vi "Teleop.vi"(10 "Match Info":T2={"Autonomous Elapsed Seconds"=0.0, "TeleOp Elapsed Seconds"=0.0, "Disabled Elapsed Seconds"=0.0, "Visited Autonomous"=FALSE, "Visited TeleOp"=FALSE, "Visited Disabled"=FALSE, "Autonomous Settings"={"Autonomous Style"=enum."Independent", "VI Refnum"=refnum}}, 11 "Call Context":T3) -> ()   [LabVIEW 2013]
doc: "This VI is called for each TeleOp packet received from the DS where the robot is not disabled. It is often used to read from the joysticks and update I/O or to update setpoints for timed control loops. It should complete and return within 20 milliseconds or it may miss DS packets."
uses:
  <vilib>/Rock Robotics/WPI/DriverStation/WPI_DriverStationDerivedRobotMode.ctl
  <vilib>/Rock Robotics/WPI/DriverStation/WPI_DriverStationMatch Info.ctl
  <vilib>/Rock Robotics/WPI/Joystick/WPI_JoystickButtonState.ctl
  <vilib>/Rock Robotics/WPI/DriverStation/WPI_DriverStationRobotMode2.ctl
  Robot Global Data.vi
  <vilib>/Rock Robotics/WPI/Joystick/WPI_JoystickGetSetRefNum.vi
  <vilib>/Rock Robotics/WPI/RobotDrive/WPI_RobotDriveGetSetRefNum.vi
  <vilib>/addons/control/pid/pid.llb/PID Control Input Filter (DBL).vi
  <vilib>/addons/control/pid/NI_PID_pid.lvlib
panel:
  in  "Drive Controls":T1
  in  "Azimuth Enabled":bool
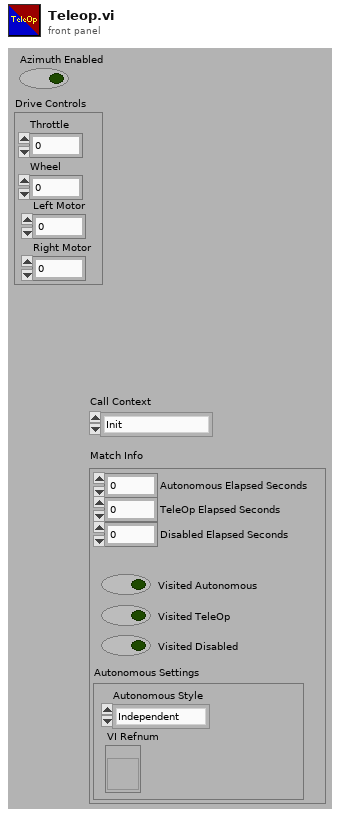
[diagram p1: front panel]
types:
  T1 = cluster{"Throttle":dbl, "Wheel":dbl, "Right Motor":dbl, "Left Motor":dbl}
  T2 = typedef "WPI_DriverStationMatch Info.ctl" = cluster{"Autonomous Elapsed Seconds":dbl, "TeleOp Elapsed Seconds":dbl, "Disabled Elapsed Seconds":dbl, "Visited Autonomous":bool, "Visited TeleOp":bool, "Visited Disabled":bool, "Autonomous Settings":cluster{"Autonomous Style":enum16{"Iterative", "Independent"}, "VI Refnum":refnum<vi>}}
  T3 = typedef "WPI_DriverStationDerivedRobotMode.ctl" = enum16{"Init", "Execute", "Stop"}
  T4 = typedef "WPI_JoystickButtonState.ctl" = cluster{"Button 1":bool, "Button 2":bool, "Button 3":bool, "Button 4":bool, "Button 5":bool, "Button 6":bool, "Button 7":bool, "Button 8":bool, "Button 9":bool, "Button 10":bool, "Button 11":bool, "Button 12":bool}
  T5 = cluster{"Driver Axes":cluster{"axis 1 (x)":dbl, "axis 2 (y)":dbl, "axis 3 (throttle)":dbl, "axis 4":dbl, "axis 5":dbl, "axis 6":dbl}, "Driver Buttons":T4, "Manipulator Axes":cluster{"axis 1 (x)":dbl, "axis 2 (y)":dbl, "axis 3 (throttle)":dbl, "axis 4":dbl, "axis 5":dbl, "axis 6":dbl}, "Manipulator Buttons":T4}
  T6 = typedef "WPI_JoystickDevRef.ctl" = cluster{"Device":T7}
  T7 = typedef "WPI_JoystickDeviceEnum.ctl" = enum16{"USB 1", "USB 2", "USB 3", "USB 4", "Kinect 1", "Kinect 2"}
  T8 = typedef "WPI_RobotDriveDevRef.ctl" = cluster{"DevStatus":errorcluster, "Motors[]":T9[], "Square Inputs":bool, "Max Output":dbl, "Isochronous":bool}
  T9 = typedef "WPI_MotorControlDeviceRef.ctl" = cluster{"DeviceStatus":errorcluster, "Type":enum16{"PWM", "CAN"}, "PWM":cluster{"Digital Module":T10, "PWM Channel":T11, "DeadBand":T12}, "CAN":cluster{"Device Number":u8, "Control Mode":T13, "Semaphore":T14, "Max Vout":dbl}, "Invert":bool, "TransformRef":T15, "InvTransformRef":T15}
  T10 = typedef "FPGA_TypedefDigitalModule.ctl" = enum16{"Digital Module 1", "Digital Module 2"}
  T11 = typedef "FPGA_DIOPWMChannel.ctl" = enum8{"PWM 1", "PWM 2", "PWM 3", "PWM 4", "PWM 5", "PWM 6", "PWM 7", "PWM 8", "PWM 9", "PWM 10", "Invalid"}
  T12 = typedef "WPI_PWMDeadband.ctl" = cluster{"Name":string, "maxPositivePwm":i32, "minPositivePwm":i32, "centerPwm":i32, "maxNegativePwm":i32, "minNegativePwm":i32, "angularRange":u16}
  T13 = typedef "WPI_CANJaguar_ControlMode.ctl" = enum8{"Percent VBus", "Current", "Speed", "Position", "Voltage"}
  T14 = typedef "Semaphore RefNum" = refnum<k1>
  T15 = typedef "WPI_PWMTransform_ConPane.ctl" = refnum<vi>
  T16 = cluster{"axis 1 (x)":dbl, "axis 2 (y)":dbl, "axis 3 (throttle)":dbl, "axis 4":dbl, "axis 5":dbl, "axis 6":dbl}
  T17 = enum16{"Wait", "Adjust Angle", "Warmup Shooter", "Fire", "Feeding", "Neutral Angle"}
  T18 = typedef "WPI_DriverStationRobotMode2.ctl" = enum16{"Autonomous Disabled", "Autonomous Enabled", "Teleop Disabled", "Teleop Enabled", "Timeout", "Finish", "Test Disabled", "Test Enabled"}
  T19 = cluster{"Quickturn_Sens_Low":dbl, "Quickturn_Sens_High":dbl, "Speedturn_Sens_Low":dbl, "Speedturn_Sens_High":dbl}
  T20 = cluster{"proportional gain (Kc)":dbl, "integral time (Ti, min)":dbl, "derivative time (Td, min)":dbl}
  T21 = typedef "Autonomous Commands.ctl" = cluster{"Load":bool, "Warmup":bool, "Low Gear":bool, "Shoot Angle":dbl, "Azimuth":bool, "Elevator":bool, "Neutral Angle":dbl, "Two Discs":bool, "Shoot":bool}
  T22 = typedef "UDP Dashboard Packet.ctl" = cluster{"Feed Angle":dbl, "Neutral Angle":dbl, "Autonomous Setpoints":T23, "Auto Shift":T24, "Elevator Angle Offset":dbl, "Potentiometer Angle":cluster{"Pot M":dbl, "Pot B":dbl}, "Shoot Setpoints":cluster{"Vision":T25, "Back Corner":T25, "Front":T25, "Front Corner":T25, "Half Court":T25, "Full Court":T25, "Pyramid":T25}, "Halo Drive":T26, "Auto Speed Constants":T27, "Shooting Delays":cluster{"Unjam On":dbl, "Unjam Off":dbl, "Flipper On":dbl, "Flipper Off":dbl, "Hopper Up":dbl}, "Left Roller Pwr":dbl, "Right Roller Pwr":dbl, "Elevator PID Gains":cluster{"proportional gain (Kc)":dbl, "integral time (Ti, min)":dbl, "derivative time (Td, min)":dbl}, "Elevator PID Output Range":cluster{"output high":dbl, "output low":dbl}, "Elevator Angle Tolerance":dbl, "Toggle Ears Delay":dbl, "Toggle Ears Distance":dbl, "Unjam Servo Angle":dbl, "Auton Steer PID gains":cluster{"proportional gain (Kc)":dbl, "integral time (Ti, min)":dbl, "derivative time (Td, min)":dbl}, "Auton Steer output range":cluster{"output high":dbl, "output low":dbl}, "Auto Reverse Speed":dbl, "Auto Stop Throttle":dbl, "Auto Stop Duration":dbl, "Spin output range":cluster{"output high":dbl, "output low":dbl}, "Spin PID gains":cluster{"proportional gain (Kc)":dbl, "integral time (Ti, min)":dbl, "derivative time (Td, min)":dbl}, "Auto-Center Line":T28, "Auton Distance PID gains Low Gear":cluster{"proportional gain (Kc)":dbl, "integral time (Ti, min)":dbl, "derivative time (Td, min)":dbl}, "Auton Distance output range":cluster{"output high":dbl, "output low":dbl}, "Auton Distance Threshold":dbl, "Auton Velocity Cutoff":dbl, "Auton Distance output range Center Line":cluster{"output high":dbl, "output low":dbl}, "Auton Distance PID gains High Gear":cluster{"proportional gain (Kc)":dbl, "integral time (Ti, min)":dbl, "derivative time (Td, min)":dbl}}
  T23 = typedef "Autonomous Setpoints.ctl" = cluster{"Shoot Angle 1":dbl, "Initial Delay":dbl, "Disc Count 1":dbl, "Shoot Time 1":dbl, "Distance 1":dbl, "Two Disc Distance 1":dbl, "Distance 2":dbl, "Two Disc Distance 2":dbl, "Distance 3":dbl, "Two Disc Distance 3":dbl, "Shoot Angle 3":dbl, "Disc Count 3":dbl, "Shoot Time 3":dbl, "Distance 4":dbl, "Two Disc Distance 4":dbl, "Low Gear":bool, "Shoot 1 Post Delay":dbl}
  T24 = typedef "Auto Shift Settings.ctl" = cluster{"Enabled":bool, "Upshift Speed":dbl, "Downshift Speed":dbl, "Upshift Throttle":dbl, "Turn Power Diff":dbl, "Motor Limit":dbl, "Encoder Limit":dbl}
  T25 = typedef "Shoot Profile.ctl" = cluster{"Pre RPM":dbl, "Main RPM":dbl, "Angle":dbl}
  T26 = typedef "Halo Drive.ctl" = cluster{"Gains":cluster{"Quickturn_Sens_Low":dbl, "Quickturn_Sens_High":dbl, "Speedturn_Sens_Low":dbl, "Speedturn_Sens_High":dbl}, "QuickTurn Const":dbl, "Loading Throttle Limit":dbl}
  T27 = typedef "Auto Speed Constants.ctl" = cluster{"Slowing Distance":dbl, "High Speed":dbl, "Rampup Time":dbl, "Low Speed":dbl, "High Speed (Reverse)":dbl}
  T28 = typedef "Autonomous Center Line Setpoints.ctl" = cluster{"Arc Turn x-axis":dbl, "Arc Turn y-axis":dbl, "Arc Turn Distance":dbl, "Distance 1":dbl, "Two Disc Distance 1":dbl, "Distance 2":dbl, "Two Disc Distance 2":dbl, "Spin Angle":dbl, "Spin Angle tolerance":dbl, "Spin y-axis":dbl, "Spin Distance":dbl, "Center Line Enabled":bool, "Distance 3":dbl, "Two Disc Distance 3":dbl, "Spin Angle 2":dbl, "Spin Angle tolerance 2":dbl, "Spin y-axis 2":dbl, "Spin Distance 2":dbl, "Shoot Angle 1":dbl, "Disc Count 1":dbl, "Shoot Time 1":dbl, "Shoot Angle 3":dbl, "Disc Count 3":dbl, "Shoot Time 3":dbl, "Low Gear":bool}
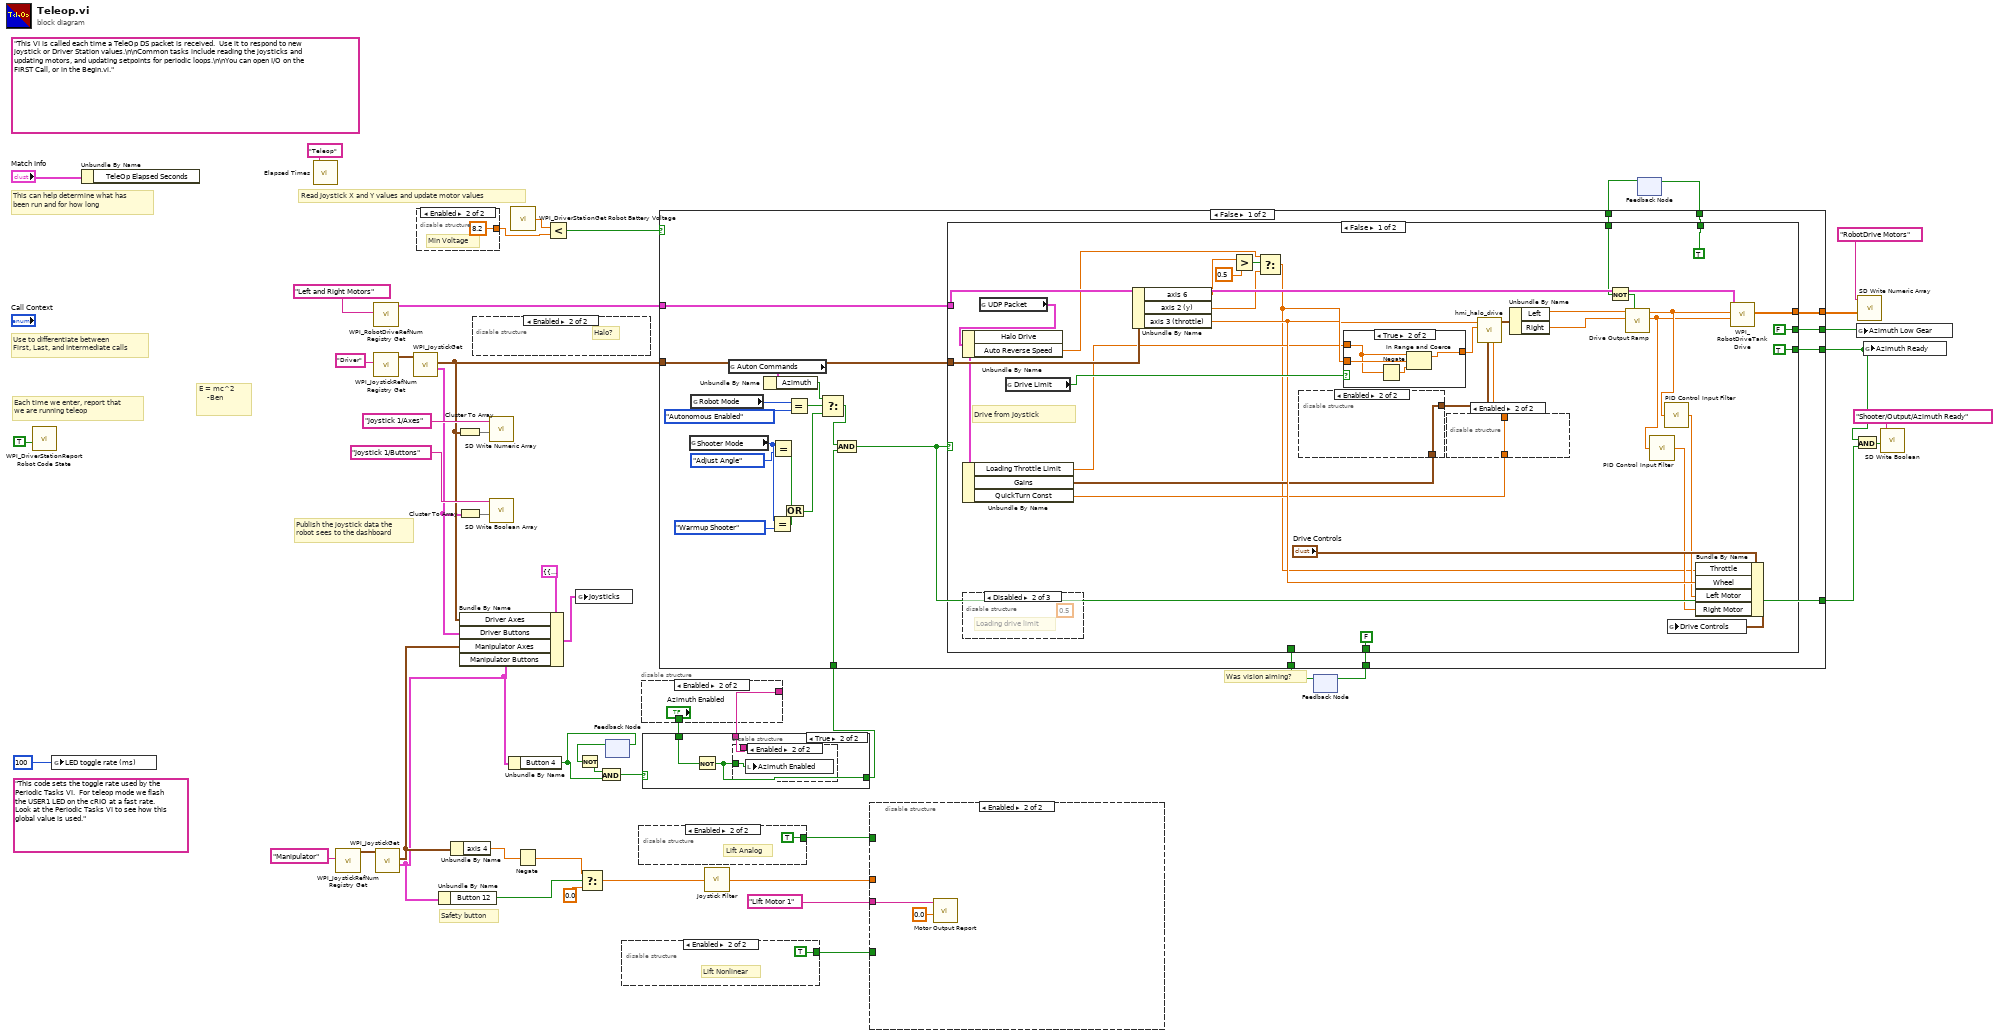
[diagram p0: block diagram]
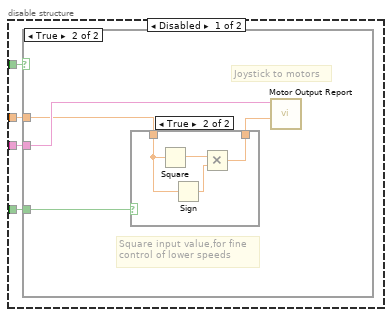
[diagram p2: hidden frame]
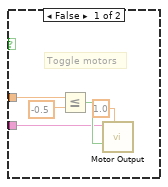
[diagram p3: hidden frame]
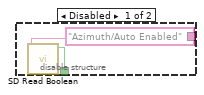
[diagram p5: hidden frame]
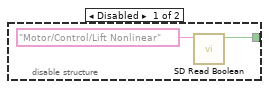
[diagram p6: hidden frame]
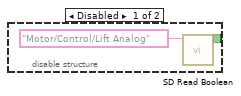
[diagram p7: hidden frame]
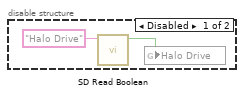
[diagram p8: hidden frame]
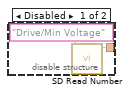
[diagram p9: hidden frame]
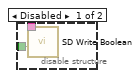
[diagram p11: hidden frame]
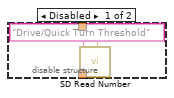
[diagram p12: hidden frame]
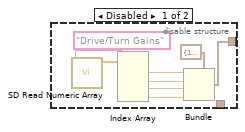
[diagram p13: hidden frame]
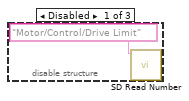
[diagram p15: hidden frame]
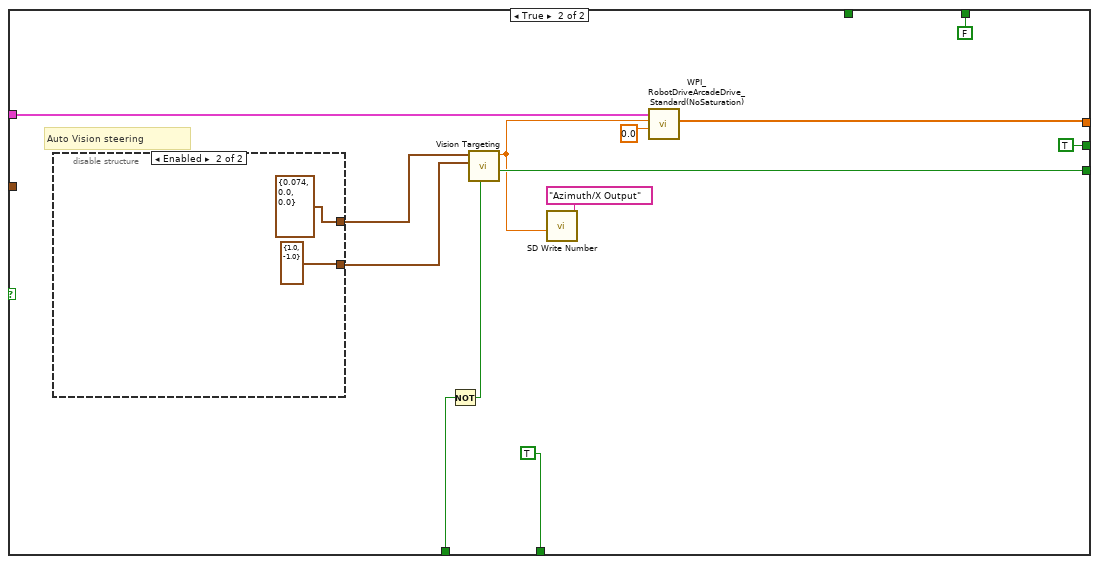
[diagram p17: hidden frame]
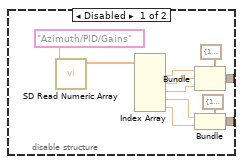
[diagram p18: hidden frame]
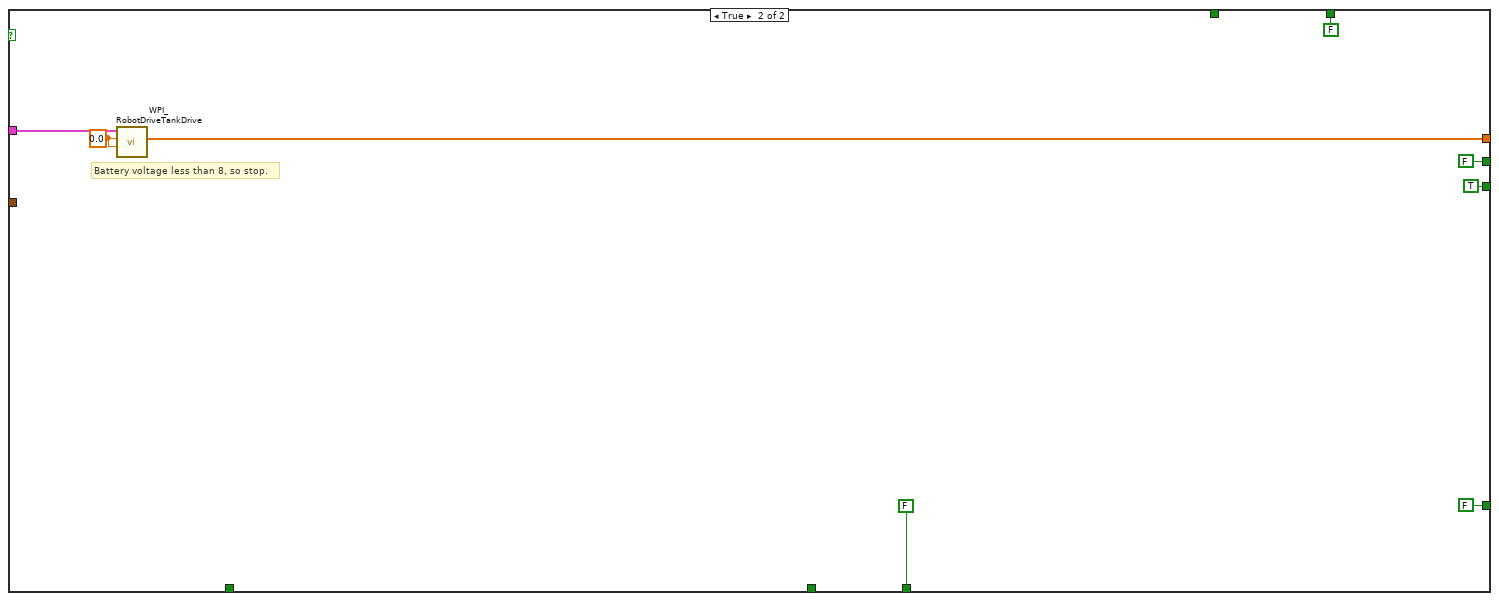
[diagram p19: hidden frame]
diagram:
  (unwired) "This code sets the toggle rate used by the Periodic Tasks VI.  For teleop mode we flash the USER1 LED on the cRIO at a fast rate.  Look at the Periodic Tasks VI to see how this global value is used."
  (unwired) "This VI is called each time a TeleOp DS packet is received.  Use it to respond to new joystick or Driver Station values.\n\nCommon tasks include reading the joysticks and updating motors, and updating setpoints for periodic loops.\n\nYou can open I/O on the FIRST Call, or in the Begin.vi."
  # "Was vision aiming?"
  # "Safety button"
  # "E = mc^2\n    -Ben"
  # "Publish the joystick data the\nrobot sees to the dashboard"
  # "Each time we enter, report that\nwe are running teleop"
  # "Use to differentiate between\nFirst, Last, and Intermediate calls"
  # "This can help determine what has\nbeen run and for how long"
  # "Read Joystick X and Y values and update motor values"
  n1 = call <vilib>:"WPI_DriverStationReport Robot Code State.vi"("TeleOp"=TRUE ("Autonomous")) -> ()  [unwired: 10 in, 1 out]
  n2 = global write "Robot Global Data.vi" "LED toggle rate (ms)"(u32 100 ("LED ms toggle rate")) -> ()
  n3 = Unbundle By Name("Match Info") -> ()  [unwired: 1 out]
  n4 = call "Elapsed Times.vi"("Call Name"="Teleop") -> ()  [unwired: 2 in, 1 out]
  n5 = call <vilib>:"WPI_JoystickRefNum Registry Get.vi"("refnum name"="Manipulator") -> ("JoystickDevRef"=w36:T6)  [unwired: 1 in, 9 out]
  n6 = call <vilib>:"WPI_RobotDriveRefNum Registry Get.vi"("refnum name"="Left and Right Motors") -> ("RobotDriveDevRef"=w39:T8)  [unwired: 1 in, 9 out]
  n7 = call <vilib>:"WPI_JoystickRefNum Registry Get.vi"("refnum name"="Driver") -> ("JoystickDevRef"=w48:T6)  [unwired: 1 in, 9 out]
  n8 = call <vilib>:"WPI_JoystickGet.vi"("JoystickDevRef"=w36) -> ("Buttons"=w4:T4, "Axes"=w24:T16)  [unwired: 1 in, 4 out]
  n9 = call <vilib>:"WPI_JoystickGet.vi"("JoystickDevRef"=w48) -> ("Buttons"=w25:T4, "Axes"=w26:T16)  [unwired: 1 in, 4 out]
  n10 = disable-structure shown="Enabled" {
    disable-tunnel: [w51 8.2 ("Numeric")] -> w20
    frame Disabled {
      n11 = call <vilib>:"SD Read Number.vi"("Name"="Drive/Min Voltage") -> ("Numeric"=w51:dbl)  [unwired: 8 in, 2 out]
    }
    frame Enabled {
      # "Min Voltage"
    }
  }
  n12 = Unbundle By Name(w4) -> ("Button 12"=w34:bool)
  n13 = Unbundle By Name(w24) -> ("axis 4"=w32:dbl)
  n14 = Cluster To Array(cluster=w26) -> (array=w43:dbl[])
  n15 = Cluster To Array(cluster=w25) -> (array=w45:bool[])
  n16 = Bundle By Name(cluster=T5 {"Driver Axes"={"axis 1 (x)"=0.0, "axis 2 (y)"=0.0, "axis 3 (throttle)"=0.0, "axis 4"=0.0, "axis 5"=0.0, "axis 6"=0.0}, "Driver Buttons"={"Button 1"=FALSE, "Button 2"=FALSE, "Button 3"=FALSE, "Button 4"=FALSE, "Button 5"=FALSE, "Button 6"=FALSE, "Button 7"=FALSE, "Button 8"=FALSE, "Button 9"=FALSE, "Button 10"=FALSE, "Button 11"=FALSE, "Button 12"=FALSE}, "Manipulator Axes"={"axis 1 (x)"=0.0, "axis 2 (y)"=0.0, "axis 3 (throttle)"=0.0, "axis 4"=0.0, "axis 5"=0.0, "axis 6"=0.0}, "Manipulator Buttons"={"Button 1"=FALSE, "Button 2"=FALSE, "Button 3"=FALSE, "Button 4"=FALSE, "Button 5"=FALSE, "Button 6"=FALSE, "Button 7"=FALSE, "Button 8"=FALSE, "Button 9"=FALSE, "Button 10"=FALSE, "Button 11"=FALSE, "Button 12"=FALSE}} ("output cluster"), "Driver Axes"=w26, "Driver Buttons"=w25, "Manipulator Axes"=w24, "Manipulator Buttons"=w4) -> (w27:T5)
  n17 = disable-structure shown="Enabled" {
    frame Disabled {
      n18 = call <vilib>:"SD Read Boolean.vi"("Name"="Halo Drive") -> ("Boolean"=w54:bool)  [unwired: 8 in, 2 out]
      n19 = global write "Robot Global Data.vi" "Halo Drive"(w54) -> ()
    }
    frame Enabled {
      # "Halo?"
    }
  }
  n20 = call <vilib>:"SD Write Numeric Array.vi"("Numeric Array"=w43, "Name"="Joystick 1/Axes") -> ()  [unwired: 8 in, 2 out]
  n21 = call <vilib>:"SD Write Boolean Array.vi"("Boolean Array"=w45, "Name"="Joystick 1/Buttons") -> ()  [unwired: 8 in, 2 out]
  n22 = Unbundle By Name(w4) -> ("Button 4"=w6:bool)
  n23 = call <vilib>:"WPI_DriverStationGet Robot Battery Voltage.vi"() -> ("robot battery voltage"=w31:dbl)  [unwired: 14 in, 1 out]
  n24 = Negate(x=w32) -> (-x=w33:dbl)
  n25 = Less?(x=w31, y=w20) -> (x < y?=w30:bool)
  n26 = global write "Robot Global Data.vi" "Joysticks"(w27) -> ()
  n27 = Select(t=w33, s=w34, f=0.0) -> (s? t:f=w23:dbl)
  n28 = feedback #1() -> (w7:bool)  [unwired: 1 in]
  n29 = Not(x=w7) -> (.not. x?=w8:bool)
  n30 = And(x=w8, y=w6) -> (x .and. y?=w5:bool)
  n31 = feedback-in #1(w6) -> ()
  n32 = disable-structure shown="Enabled" {
    disable-tunnel: [w56 TRUE ("Boolean")] -> w18
    frame Disabled {
      n33 = call <vilib>:"SD Read Boolean.vi"("Name"="Motor/Control/Lift Nonlinear") -> ("Boolean"=w56:bool)  [unwired: 8 in, 2 out]
    }
    frame Enabled {
      # "Lift Nonlinear"
    }
  }
  n34 = disable-structure shown="Enabled" {
    disable-tunnel: [w59 TRUE ("Boolean")] -> w28
    frame Disabled {
      n35 = call <vilib>:"SD Read Boolean.vi"("Name"="Motor/Control/Lift Analog") -> ("Boolean"=w59:bool)  [unwired: 8 in, 2 out]
    }
    frame Enabled {
      # "Lift Analog"
    }
  }
  n36 = disable-structure shown="Enabled" {
    disable-tunnel: [w63 _] -> w10
    disable-tunnel: [w62 "Azimuth Enabled"] -> w9
    frame Disabled {
      w63 = "Azimuth/Auto Enabled" ("Name")
      n37 = call <vilib>:"SD Read Boolean.vi"("Name"=w63) -> ("Boolean"=w62:bool)  [unwired: 8 in, 2 out]
    }
    frame Enabled {
    }
  }
  n38 = case shown="True" w5 {
    tunnel: w9 -> [w65 w68]
    tunnel: w10 -> [_ w67]
    tunnel: [w65 w66] -> w3
    frame False {
    }
    frame True {
      n39 = Not(x=w68) -> (.not. x?=w66:bool)
      n40 = disable-structure shown="Enabled" {
        disable-tunnel: w67 -> [w70 _]
        disable-tunnel: w66 -> [w69 w71]
        frame Disabled {
          n41 = call <vilib>:"SD Write Boolean.vi"("Boolean"=w69, "Name"=w70) -> ()  [unwired: 8 in, 2 out]
        }
        frame Enabled {
          n42 = local write "Azimuth Enabled"(w71) -> ()
        }
      }
    }
  }
  n43 = call "Joystick Filter.vi"("In"=w23) -> ("Out"=w22:dbl)
  n44 = disable-structure shown="Enabled" {
    disable-tunnel: "Lift Motor 1" ("refnum name") -> [w75 w91]
    disable-tunnel: w28 -> [w74 _]
    disable-tunnel: w22 -> [w73 _]
    disable-tunnel: w18 -> [w72 _]
    frame Disabled {
      n45 = case shown="True" w74 {
        tunnel: w73 -> [w78 w82]
        tunnel: w75 -> [w77 w84]
        tunnel: w72 -> [_ w81]
        frame False {
          # "Toggle motors"
          n46 = Less Or Equal?(x=w78, y=-0.5) -> (x <= y?=w79:bool)
          n47 = call "Motor Output.vi"("Max Power"=1.0, "Backward"=w79, "Motor refnum name"=w77) -> ()  [unwired: 8 in, 1 out]
        }
        frame True {
          # "Square input value,for fine\ncontrol of lower speeds"
          # "Joystick to motors"
          n48 = case shown="True" w81 {
            tunnel: [w85 w87] -> w83
            tunnel: w82 -> [w85 w86]
            frame False {
              # "linear"
            }
            frame True {
              n49 = Square(x=w86) -> (x^2=w88:dbl)
              n50 = Sign(1:w86) -> (0:w89:dbl)
              n51 = Multiply(x=w88, y=w89) -> (x*y=w87:dbl)
            }
          }
          n52 = call "Motor Output Report.vi"("Motor Speed"=w83, "Motor refnum name"=w84) -> ()  [unwired: 9 in, 1 out]
        }
      }
    }
    frame Enabled {
      n53 = call "Motor Output Report.vi"("Motor Speed"=0.0, "Motor refnum name"=w91) -> ()  [unwired: 9 in, 1 out]
    }
  }
  n54 = feedback #2() -> (w16:bool)  [unwired: 1 in]
  n55 = feedback #3() -> (w1:bool)  [unwired: 1 in]
  n56 = case shown="False" w30 {
    tunnel: [w114 w199] -> w40
    tunnel: w39 -> [w113 w200]
    tunnel: w26 -> [w112 _]
    tunnel: [w108 TRUE ("Azimuth Ready")] -> w12
    tunnel: [w107 FALSE ("Azimuth Ready")] -> w17
    tunnel: w16 -> [w106 _]
    tunnel: [w105 FALSE ("Azimuth Ready")] -> w14
    tunnel: [w97 FALSE] -> w11
    tunnel: w3 -> [w94 _]
    tunnel: [w93 FALSE ("Azimuth Ready")] -> w2
    tunnel: w1 -> [w92 _]
    frame False {
      n57 = global read "Robot Global Data.vi" "Shooter Mode"() -> (w109:T17)
      n58 = global read "Robot Global Data.vi" "Robot Mode"() -> (w100:T18)
      n59 = global read "Robot Global Data.vi" "Auton Commands"() -> (w102:T21)
      n60 = Unbundle By Name(w102) -> ("Azimuth"=w101:bool)
      n61 = Equal?(x=w109, y=T17."Warmup Shooter" ("Shooter Mode")) -> (x = y?=w111:bool)
      n62 = Equal?(x=w109, y=T17."Adjust Angle" ("Shooter Mode")) -> (x = y?=w110:bool)
      n63 = Or(x=w110, y=w111) -> (x .or. y?=w103:bool)
      n64 = Equal?(x=w100, y=WPI_DriverStationRobotMode2."Autonomous Enabled") -> (x = y?=w98:bool)
      n65 = Select(t=w101, s=w98, f=w103) -> (s? t:f=w104:bool)
      n66 = And(x=w104, y=w94) -> (x .and. y?=w97:bool)
      n67 = case shown="False" w97 {
        tunnel: [w148 w177] -> w114
        tunnel: w113 -> [w147 w179]
        tunnel: w112 -> [w146 _]
        tunnel: [TRUE ("Azimuth Ready") w174] -> w108
        tunnel: [FALSE ("Azimuth Ready") TRUE ("Azimuth Ready")] -> w107
        tunnel: w106 -> [_ w172]
        tunnel: [FALSE ("Azimuth Ready") TRUE ("Azimuth Ready")] -> w105
        tunnel: [TRUE ("Azimuth Ready") FALSE ("Azimuth Ready")] -> w93
        tunnel: w92 -> [w137 _]
        frame False {
          # "Drive from Joystick"
          n68 = disable-structure shown="Disabled" {
            frame Disabled {
              n69 = call <vilib>:"SD Read Number.vi"("Name"="Motor/Control/Drive Limit") -> ()  [unwired: 8 in, 3 out]
            }
            frame Disabled {
              (unwired) 0.5 ("Numeric")
              # "Loading drive limit"
            }
            frame Enabled {
            }
          }
          n70 = global read "Robot Global Data.vi" "UDP Packet"() -> (w133:T22)
          n71 = Unbundle By Name(w133) -> ("Halo Drive"=w132:T26, "Auto Reverse Speed"=w116:dbl)
          n72 = Unbundle By Name(w132) -> ("Loading Throttle Limit"=w134:dbl, "Gains"=w136:T19, "QuickTurn Const"=w135:dbl)
          n73 = global read "Robot Global Data.vi" "Drive Limit"() -> (w145:bool)
          n74 = Unbundle By Name(w146) -> ("axis 6"=w115:dbl, "axis 2 (y)"=w118:dbl, "axis 3 (throttle)"=w144:dbl)
          n75 = Greater?(x=w115, y=0.5) -> (0:w119:bool)
          n76 = Select(t=w116, s=w119, f=w118) -> (s? t:f=w117:dbl)
          n77 = disable-structure shown="Enabled" {
            disable-tunnel: [w152 w160] -> w130
            disable-tunnel: w136 -> [_ w160]
            frame Disabled {
              n78 = call <vilib>:"SD Read Numeric Array.vi"("Name"="Drive/Turn Gains") -> ("Numeric Array"=w159:dbl[])  [unwired: 8 in, 2 out]
              n79 = Index Array(array=w159) -> (element #1=w156:dbl, element #2=w155:dbl, element #3=w154:dbl, element #4=w153:dbl)  [unwired: 4 in]
              n80 = Bundle(cluster=T19 {"Quickturn_Sens_Low"=1.2, "Quickturn_Sens_High"=1.0, "Speedturn_Sens_Low"=1.5, "Speedturn_Sens_High"=1.7} ("Turn Gains"), "Quickturn_Sens_Low"=w156, "Quickturn_Sens_High"=w155, "Speedturn_Sens_Low"=w154, "Speedturn_Sens_High"=w153) -> (w152:T19)
            }
            frame Enabled {
            }
          }
          n81 = case shown="True" w145 {
            tunnel: w144 -> [w161 w165]
            tunnel: [w161 w162] -> w131
            tunnel: w134 -> [_ w163]
            frame False {
            }
            frame True {
              n82 = Negate(x=w163) -> (-x=w164:dbl)
              n83 = In Range and Coerce(upper limit=w163, x=w165, lower limit=w164) -> (coerced(x)=w162:dbl)  [unwired: 1 out]
            }
          }
          n84 = disable-structure shown="Enabled" {
            disable-tunnel: [w149 w151] -> w129
            disable-tunnel: w135 -> [_ w151]
            frame Disabled {
              n85 = call <vilib>:"SD Read Number.vi"("Name"="Drive/Quick Turn Threshold") -> ("Numeric"=w149:dbl)  [unwired: 8 in, 2 out]
            }
            frame Enabled {
            }
          }
          n86 = call "hmi_halo_drive.vi"("QuickTurn Const"=w129, "Turn Gains"=w130, "Wheel"=w131, "Throttle"=w117) -> ("Drive Data"=w127:cluster{"Left":dbl, "Right":dbl})  [unwired: 7 in]
          n87 = Unbundle By Name(w127) -> ("Left"=w125:dbl, "Right"=w126:dbl)
          n88 = Not(x=w137) -> (.not. x?=w128:bool)
          n89 = call "Drive Output Ramp.vi"("reinitialize?"=w128, "Right"=w126, "Left"=w125) -> ("Right Output"=w121:dbl, "Left Output"=w122:dbl)  [unwired: 7 in]
          n90 = call-poly <vilib>:"PID Control Input Filter.vi"("input"=w121) -> ("output"=w123:dbl)  [unwired: 4 in]
          n91 = call-poly <vilib>:"PID Control Input Filter.vi"("input"=w122) -> ("output"=w124:dbl)  [unwired: 4 in]
          n92 = Bundle By Name(cluster="Drive Controls", "Throttle"=w117, "Wheel"=w144, "Left Motor"=w124, "Right Motor"=w123) -> (w142:T1)
          n93 = global write "Robot Global Data.vi" "Drive Controls"(w142) -> ()
          n94 = call <vilib>:"WPI_RobotDriveTankDrive.vi"("Right axis value"=w121, "Left axis value"=w122, "RobotDriveDevRef"=w147) -> ("Motor Values"=w148:dbl[])  [unwired: 6 in, 2 out]
        }
        frame True {
          # "Auto Vision steering"
          n95 = disable-structure shown="Enabled" {
            disable-tunnel: [w183 T20 {"proportional gain (Kc)"=0.074, "integral time (Ti, min)"=0.0, "derivative time (Td, min)"=0.0} ("PID gains")] -> w176
            disable-tunnel: [w182 cluster{"output high":dbl, "output low":dbl} {"output high"=1.0, "output low"=-1.0} ("output range")] -> w175
            frame Disabled {
              n96 = call <vilib>:"SD Read Numeric Array.vi"("Name"="Azimuth/PID/Gains") -> ("Numeric Array"=w188:dbl[])  [unwired: 8 in, 2 out]
              n97 = Index Array(array=w188) -> (element #1=w187:dbl, element #2=w186:dbl, element #3=w185:dbl, element #4=w181:dbl, element #5=w180:dbl)  [unwired: 5 in]
              n98 = Bundle(cluster=T20 {"proportional gain (Kc)"=1.0, "integral time (Ti, min)"=0.01, "derivative time (Td, min)"=0.0} ("PID gains"), "proportional gain (Kc)"=w187, "integral time (Ti, min)"=w186, "derivative time (Td, min)"=w185) -> (w183:T20)
              n99 = Bundle(cluster=cluster{"output high":dbl, "output low":dbl} {"output high"=100.0, "output low"=-100.0} ("output range"), "output high"=w181, "output low"=w180) -> (w182:cluster{"output high":dbl, "output low":dbl})
            }
            frame Enabled {
            }
          }
          n100 = Not(x=w172) -> (.not. x?=w171:bool)
          n101 = call "Vision Targeting.vi"("reinitialize?"=w171, "output range"=w175, "PID gains"=w176) -> ("Azimuth Ready"=w174:bool, "X Axis output"=w169:dbl)  [unwired: 7 in]
          n102 = call <vilib>:"SD Write Number.vi"("Numeric"=w169, "Name"="Azimuth/X Output") -> ()  [unwired: 8 in, 2 out]
          n103 = call <vilib>:"WPI_RobotDriveArcadeDrive_Standard(NoSaturation).vi"("Y axis value"=0.0, "X axis value"=w169, "RobotDriveDevRef"=w179) -> ("Motor Values"=w177:dbl[])  [unwired: 1 in, 7 out]
        }
      }
    }
    frame True {
      w198 = 0.0 ("Left axis value")
      # "Battery voltage less than 8, so stop."
      n104 = call <vilib>:"WPI_RobotDriveTankDrive.vi"("Right axis value"=w198, "Left axis value"=w198, "RobotDriveDevRef"=w200) -> ("Motor Values"=w199:dbl[])  [unwired: 6 in, 2 out]
    }
  }
  n105 = feedback-in #2(w17) -> ()
  n106 = feedback-in #3(w2) -> ()
  n107 = And(x=w12, y=w11) -> (x .and. y?=w13:bool)
  n108 = global write "Robot Global Data.vi" "Azimuth Low Gear"(w14) -> ()
  n109 = call <vilib>:"SD Write Numeric Array.vi"("Numeric Array"=w40, "Name"="RobotDrive Motors") -> ()  [unwired: 8 in, 2 out]
  n110 = global write "Robot Global Data.vi" "Azimuth Ready"(w12) -> ()
  n111 = call <vilib>:"SD Write Boolean.vi"("Boolean"=w13, "Name"="Shooter/Output/Azimuth Ready") -> ()  [unwired: 8 in, 2 out]
